vi "new results.vi"(8 "error in (no error)":errorcluster, 9 "Results In":refnum<class "Analyze Results Base.lvclass">[](array[class]), 10 "Parameters":refnum<class "Analyze Parameter Base.lvclass">[](array[class]), 11 "Launch IMAQ Display in":refnum<class "HIJ Vision Camera App.lvclass">) -> (0 "error out":errorcluster, 3 "Launch IMAQ Display out":refnum<class "HIJ Vision Camera App.lvclass">)   [LabVIEW 2014, in "HIJ Vision Camera App.lvlib" / "HIJ Vision Camera App.lvclass"]
uses:
  HIJ Vision Camera App.lvclass
  Results and Overlays/Results Base/Analyze Results Base.lvclass
  Analyze Parameter/Analyze Parameter Base/Analyze Parameter Base.lvclass
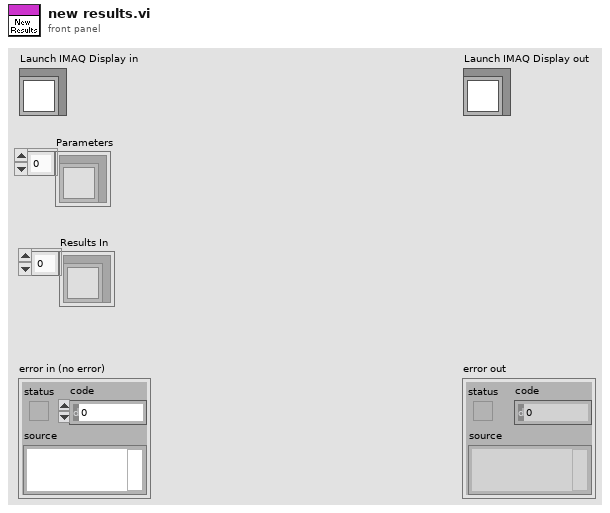
[diagram p1: front panel]
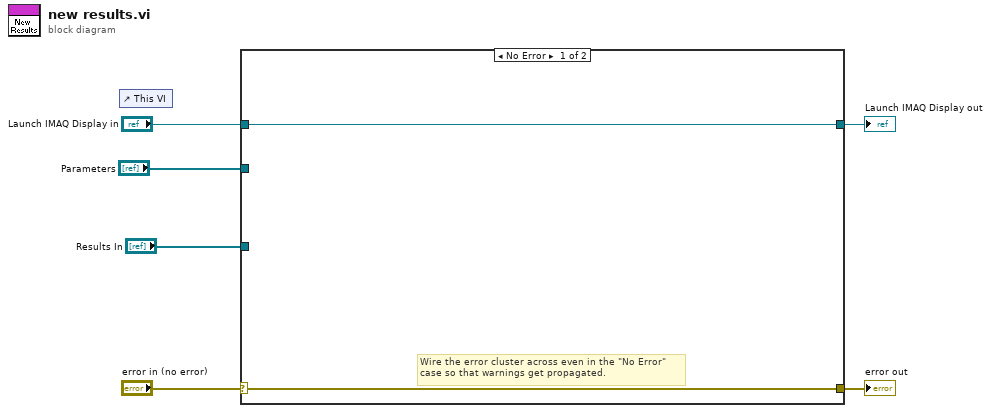
[diagram p0: block diagram]
diagram:
  n1 = control-ref of="This VI"() -> ()  [unwired: 1 out]
  n2 = case shown="No Error" "error in (no error)" {
    selector: "error in (no error)" -> [w7 w10]
    tunnel: [w7 w10] -> w5
    tunnel: [w8 w9] -> w3
    tunnel: "Launch IMAQ Display in" -> [w8 w9]
    tunnel: "Parameters" -> [_ _]
    tunnel: "Results In" -> [_ _]
    frame No Error {
      # "Wire the error cluster across even in the \"No Error\"\ncase so that warnings get propagated."
    }
    frame Error {
    }
  }
  "error out" <- w5
  "Launch IMAQ Display out" <- w3
